vi "Build Command Line Arguments.vi"(10 "Arguments":string[](array[string]), 11 "Executable File Name":string="Revert to Scan Mode.exe") -> (3 "Command Line":string)   [LabVIEW 2021, in "CANOpen Addon System Explorer.lvlib"]
uses:
  CANOpen Addon System Explorer.lvlib
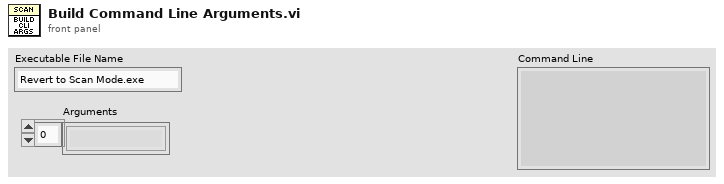
[diagram p1: front panel]
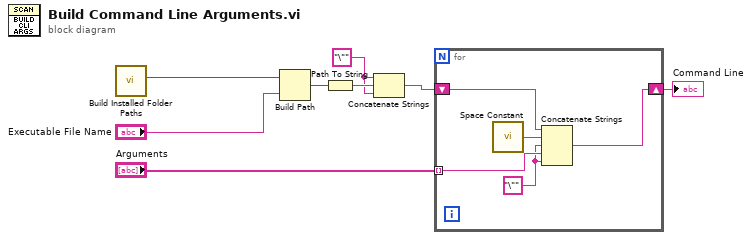
[diagram p0: block diagram]
diagram:
  w2 = "\""
  n1 = call "Build Installed Folder Paths.vi"() -> ("Application Folder Path"=w1:path)  [unwired: 10 in, 1 out]
  n2 = Build Path(base path=w1, name or relative path="Executable File Name") -> (appended path=w6:path)
  n3 = Path To String(path=w6) -> (string=w8:string)
  n4 = Concatenate Strings(w2, w8, w2) -> (w4:string)
  n5 = for {
    tunnel: "Arguments" -> [w11] mode=indexing
    shift-right: [w12] -> w3
    shift-left: w4 -> [w13]
    w10 = "\""
    n6 = call <vilib>:"Space Constant.vi"() -> ("String"=w9:string)
    n7 = Concatenate Strings(w13, w9, w10, w11, w10) -> (w12:string)
  }
  "Command Line" <- w3
